vi "LED SegmentControl.vi"(8 "error in":errorcluster, 10 "notifier in":refnum<notifier>) -> (0 "error out":errorcluster)   [LabVIEW 2010, in "lib1299.lvlib"]
doc: "This VI serves to write values to the LCD segment display using the seg file.\n\nInputs:\nNotifier In - notifier reference"
uses:
  lib1299.lvlib
  TYP_LEDCommand.ctl
  Styx/lvstyx/Write/lvstyx_write_path_int.vi
  TYP_LEDSegNotifier.ctl
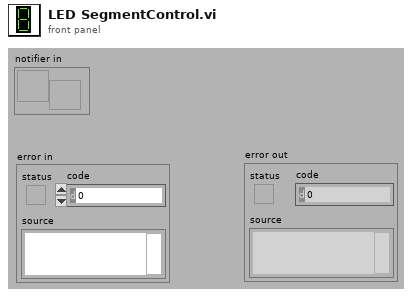
[diagram p1: front panel]
types:
  T1 = typedef "lib1299.lvlib/TYP_LEDCommand.ctl" = enum16{"Init", "Go ACQ", "Go XFR", "Manual", "Stop", "Exit"}
  T2 = typedef "lib1299.lvlib/TYP_LEDSegNotifier.ctl" = cluster{"notification":T1, "Data":i32}
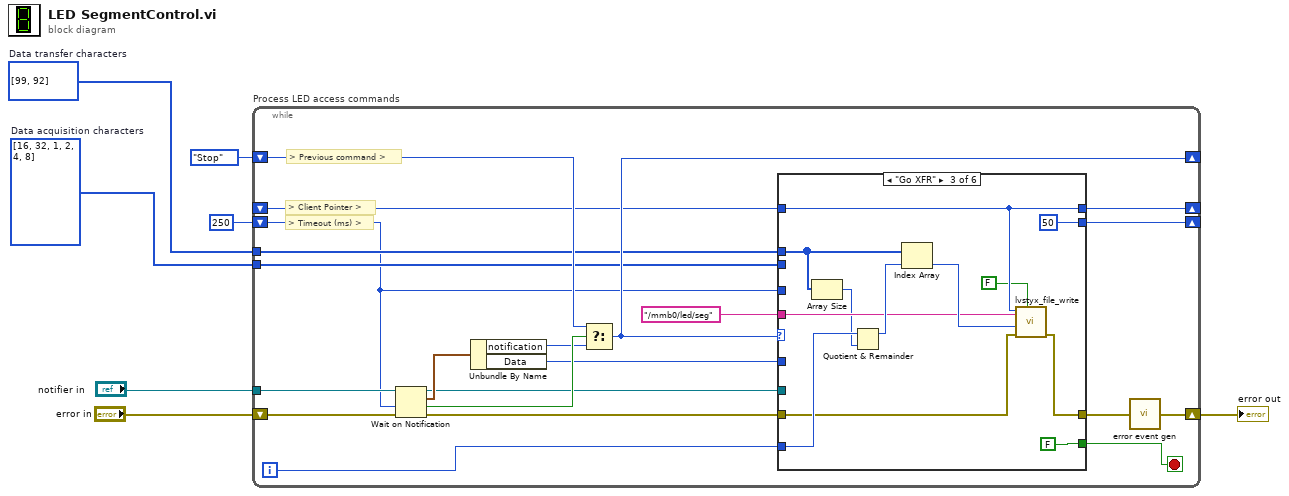
[diagram p0: block diagram]
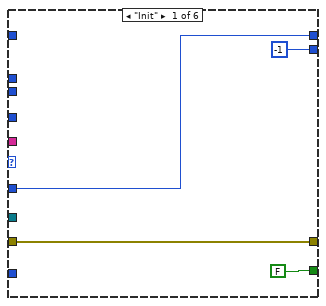
[diagram p2: hidden frame]
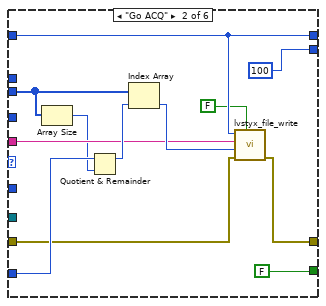
[diagram p3: hidden frame]
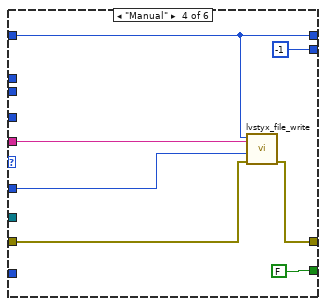
[diagram p4: hidden frame]
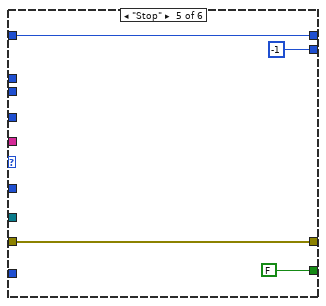
[diagram p5: hidden frame]
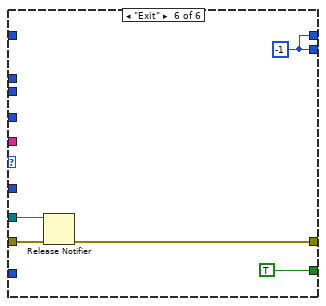
[diagram p6: hidden frame]
diagram:
  w6 = i32[] [16, 32, 1, 2, 4, 8]  # Data acquisition characters
  w7 = i32[] [99, 92]  # Data transfer characters
  n1 = while "Process LED access commands" {
    tunnel: "notifier in" -> [w28]
    shift-right: [w25] -> _
    shift-left: TYP_LEDCommand."Stop" ("Enum") -> [w26]
    tunnel: w7 -> [w23]
    tunnel: w6 -> [w22]
    shift-right: [w20] -> _
    shift-left: _ -> [w21]
    shift-right: [w12] -> _
    shift-left: 250 ("timeout in ms (-1)") -> [w17]
    shift-right: [w9] -> w1
    shift-left: "error in" -> [w24]
    i -> [w18]
    stop <- w19 stop-if-true
    # "> Timeout (ms) >"
    # "> Client Pointer >"
    # "> Previous command >"
    n2 = Wait on Notification(notifier=w28, timeout in ms (-1)=w17, error in (no error)=w24) -> (notifier out=w13:refnum<notifier>, notification=w16:T2, timed out?=w27:bool, error out=w11:errorcluster)  [unwired: 1 in]
    n3 = Unbundle By Name(w16) -> ("notification"=w15:T1, "Data"=w14:i32)
    n4 = Select(t=w26, s=w27, f=w15) -> (s? t:f=w25:T1)
    n5 = case shown="\"Go XFR\"" w25 {
      tunnel: w23 -> [_ _ w47 _ _ _]
      tunnel: w22 -> [_ w35 _ _ _ _]
      tunnel: w21 -> [_ w40 w51 w61 w66 _]
      tunnel: w14 -> [w32 _ _ w57 _ _]
      tunnel: [w32 w40 w51 w61 w66 w68] -> w20
      tunnel: [FALSE FALSE FALSE FALSE FALSE TRUE] -> w19
      tunnel: w18 -> [_ w43 w55 _ _ _]
      tunnel: w17 -> [_ _ _ _ _ _]
      tunnel: [i64 -1 ("int64") 100 ("timeout in ms (-1)") 50 ("timeout in ms (-1)") -1 ("timeout in ms (-1)") -1 ("timeout in ms (-1)") w68] -> w12
      tunnel: w13 -> [_ _ _ _ _ w71]
      tunnel: w11 -> [w29 w38 w50 w60 w64 w70]
      tunnel: [w29 w37 w49 w59 w64 w69] -> w10
      tunnel: "/mmb0/led/seg" ("path") -> [_ w36 w48 w58 _ _]
      frame "Init" {
      }
      frame "Go ACQ" {
        n6 = Array Size(array=w35) -> (size(s)=w34:i32)
        n7 = Quotient & Remainder(x=w43, y=w34) -> (x-y*floor(x/y)=w42:i32)  [unwired: 1 out]
        n8 = Index Array(array=w35, index=w42) -> (element=w39:i32)
        n9 = call-poly "lvstyx_file_write.vi"("Log? (T)"=FALSE, "error in (no error)"=w38, "int64"=w39, "path"=w36, "client ptr"=w40) -> ("error out"=w37:errorcluster)  [unwired: 5 in, 1 out]
      }
      frame "Go XFR" {
        n10 = Array Size(array=w47) -> (size(s)=w46:i32)
        n11 = Quotient & Remainder(x=w55, y=w46) -> (x-y*floor(x/y)=w54:i32)  [unwired: 1 out]
        n12 = Index Array(array=w47, index=w54) -> (element=w52:i32)
        n13 = call-poly "lvstyx_file_write.vi"("Log? (T)"=FALSE, "error in (no error)"=w50, "int64"=w52, "path"=w48, "client ptr"=w51) -> ("error out"=w49:errorcluster)  [unwired: 5 in, 1 out]
      }
      frame "Manual" {
        n14 = call-poly "lvstyx_file_write.vi"("error in (no error)"=w60, "int64"=w57, "path"=w58, "client ptr"=w61) -> ("error out"=w59:errorcluster)  [unwired: 6 in, 1 out]
      }
      frame "Stop" {
      }
      frame "Exit" {
        w68 = i64 -1 ("int64")
        n15 = Release Notifier(notifier=w71, error in (no error)=w70) -> (error out=w69:errorcluster)  [unwired: 1 in, 2 out]
      }
    }
    n16 = call "error event gen.vi"("error in (no error)"=w10) -> ("error out"=w9:errorcluster)  [unwired: 1 out]
  }
  "error out" <- w1
